vi "Call Acquire.vi"(6 "Diagnostics Queue in":refnum<queue>, 7 "Host Resources":T11, 8 "error in (no error)":errorcluster, 11 "Hardware Configuration in":T2) -> (0 "error out":errorcluster, 2 "Acquired Data":T1, 3 "Hardware Configuration out":T2)   [LabVIEW 2021, in "Acquisition.lvlib"]
doc: "Call the Acquire API for the active plugin."
uses:
  Acquisition.lvlib
  API Call.ctl
  support/Message Queue/Message Cluster.ctl
  support/Message Queue/Message Queue.lvlib
  Host Software Package.ctl
  Host IO Resource.ctl
  Host Resources.ctl
  IO Device.ctl
  Sensor Type.ctl
  Channel Settings.ctl
  Interval Timer/Interval Length.ctl
  Interval Timer/Interval Timer.lvlib
  Interval Timer/Repeat Interval.ctl
  Interval Timer/Interval Token.ctl
  IO API.ctl
  IO Context.ctl
  Hardware Configuration.ctl
  Acquired Data.ctl
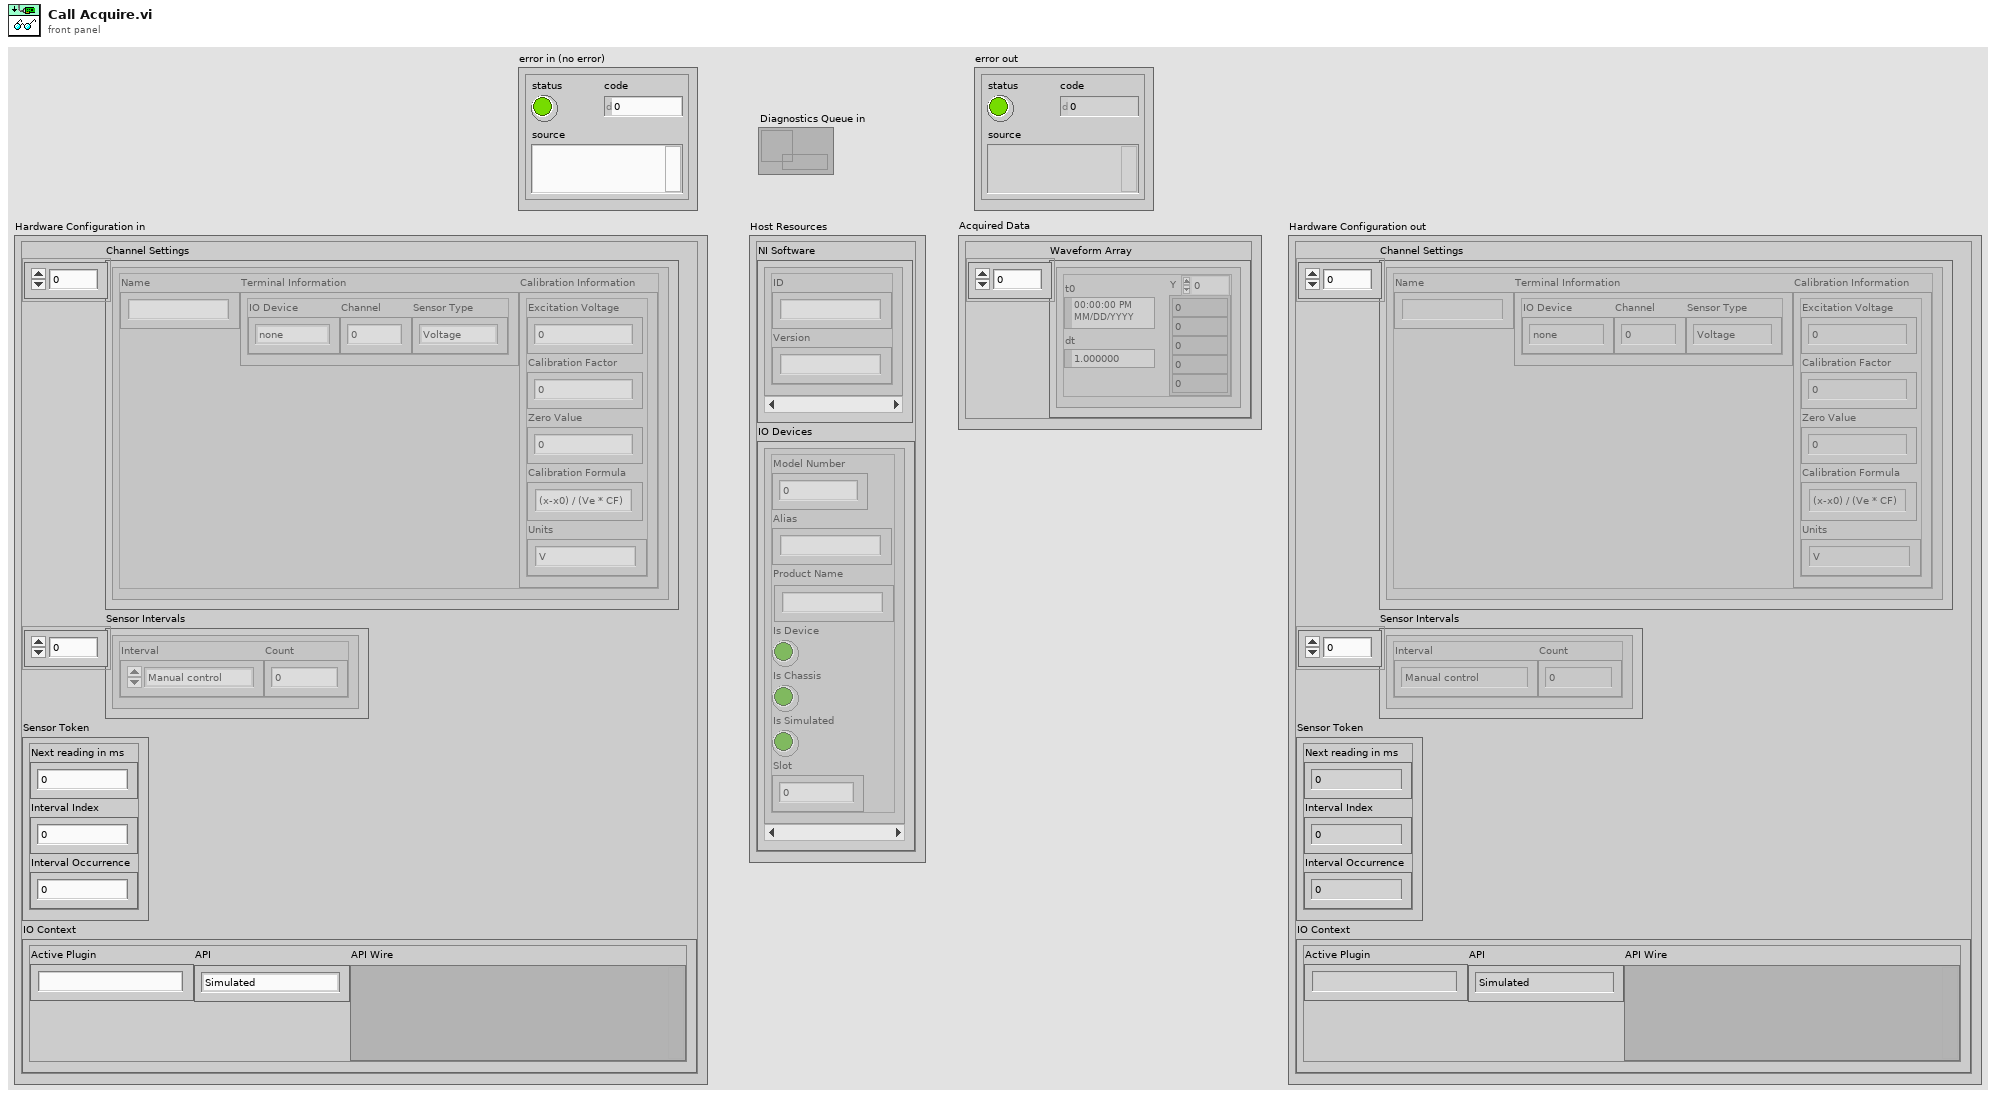
[diagram p1: front panel]
types:
  T1 = typedef "Acquisition.lvlib/Acquired Data.ctl" = cluster{"Waveform Array":waveform(dbl)[]}
  T2 = typedef "Acquisition.lvlib/Hardware Configuration.ctl" = cluster{"Channel Settings":T3[], "Sensor Intervals":T6[], "Sensor Token":T8, "IO Context":T9}
  T3 = typedef "Acquisition.lvlib/Channel Settings.ctl" = cluster{"Name":string, "Terminal Information":cluster{"IO Device":T4, "Channel":i32, "Sensor Type":T5}, "Calibration Information":cluster{"Excitation Voltage":dbl, "Calibration Factor":dbl, "Zero Value":dbl, "Calibration Formula":string, "Units":string}}
  T4 = typedef "Acquisition.lvlib/IO Device.ctl" = enum16{"none", "9219", "9401"}
  T5 = typedef "Acquisition.lvlib/Sensor Type.ctl" = enum16{"Voltage", "Load", "Pressure", "Encoder"}
  T6 = typedef "Interval Timer.lvlib/Repeat Interval.ctl" = cluster{"Interval":T7, "Count":i32}
  T7 = typedef "Interval Timer.lvlib/Interval Length.ctl" = enum16{"Manual control", "1 second", "10 seconds", "30 seconds", "60 seconds", "600 seconds", "1200 seconds", "3600 seconds"}
  T8 = typedef "Interval Timer.lvlib/Interval Token.ctl" = cluster{"Next reading in ms":u32, "Interval Index":i32, "Interval Occurrence":i32}
  T9 = typedef "Acquisition.lvlib/IO Context.ctl" = cluster{"Active Plugin":string, "API":T10, "API Wire":variant}
  T10 = typedef "Acquisition.lvlib/IO API.ctl" = enum16{"Simulated", "DAQmx"}
  T11 = typedef "Acquisition.lvlib/Host Resources.ctl" = cluster{"NI Software":T12[], "IO Devices":T13[]}
  T12 = typedef "Acquisition.lvlib/Host Software Package.ctl" = cluster{"ID":string, "Version":string}
  T13 = typedef "Acquisition.lvlib/Host IO Resource.ctl" = cluster{"Model Number":u32, "Alias":string, "Product Name":string, "Is Device":bool, "Is Chassis":bool, "Is Simulated":bool, "Slot":i32}
  T14 = typedef "Acquisition.lvlib/API Call.ctl" = enum16{"On Start", "On Acquire", "On Stop"}
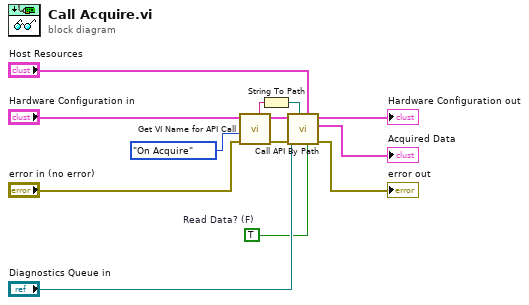
[diagram p0: block diagram]
diagram:
  w2 = TRUE  # Read Data? (F)
  n1 = call "Get VI Name for API Call.vi"("error in"="error in (no error)", "API Call"=API_Call."On Acquire", "Hardware Configuration in"="Hardware Configuration in") -> ("error out"=w6:errorcluster, "Hardware Configuration out"=w3:T2, "VI Name"=w8:string)  [unwired: 6 in]
  n2 = String To Path(string=w8) -> (path=w9:path)
  n3 = call "Call API By Path.vi"("Read Data? (F)"=w2, "Host Resources"="Host Resources", "vi path"=w9, "error in"=w6, "Diagnostics Queue"="Diagnostics Queue in", "Hardware Configuration in"=w3) -> ("error out"=→"error out":errorcluster, "Acquired Data"=→"Acquired Data":T1, "Hardware Configuration out"=→"Hardware Configuration out":T2)  [unwired: 3 in]
